vi "RP Read Subset.vi"(6 "Mode":T2=enum."Digitizer", 8 "Error In":errorcluster, 9 "Parameters":T1={"Ranges"=[20.0, 20.0], "Output frequency 1"=50000.0, "Output frequency 2"=50000.0, "Trigger offset"=-100000, "Post-trigger samples"=11534336, "Desimation rate"=125} {"Post-trigger samples" format="0x%x (%d)"; "Trigger offset" format="0x%x (%d)"; "Output frequency 2" format="%#_6p"; "Output frequency 1" format="%#_6p"}, 11 "connection ID":refnum<k5>) -> (0 "Error Out":errorcluster, 1 "Record start pos":u32=1, 2 "Data stream":string, 3 "connection ID out":refnum<k5>)   [LabVIEW 2015]
uses:
  Mode.ctl
  Red Pitaya Parameters.ctl
  RP Command.ctl
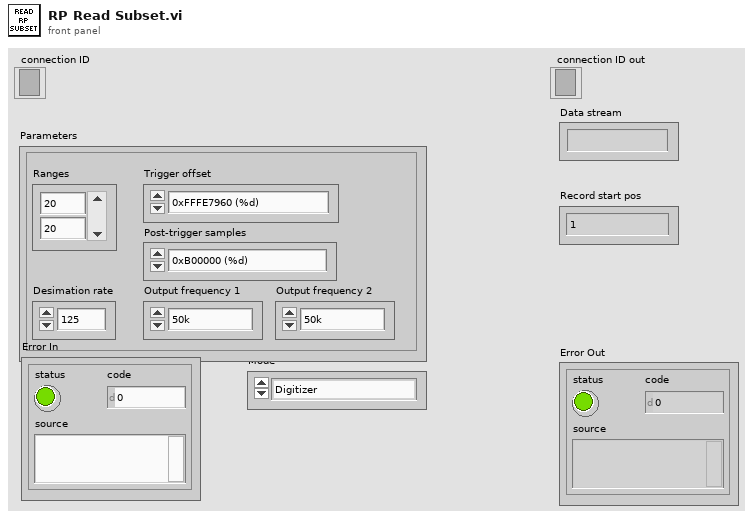
[diagram p1: front panel]
types:
  T1 = typedef "Red Pitaya Parameters.ctl" = cluster{"Ranges":dbl[], "Output frequency 1":dbl, "Output frequency 2":dbl, "Trigger offset":i32, "Post-trigger samples":u64, "Desimation rate":u64}
  T2 = typedef "Mode.ctl" = enum16{"Filter", "Lockin test", "Snapshot test", "Digitizer"}
  T3 = typedef "RP Command.ctl" = enum16{"Set frequency", "Arm and get data", "Stop server", "Get status", "Get temperature", "Set decimation", "Arm", "Software trigger", "Get whole buffer", "Get chunk", "System call", "Get config", "Set config"}
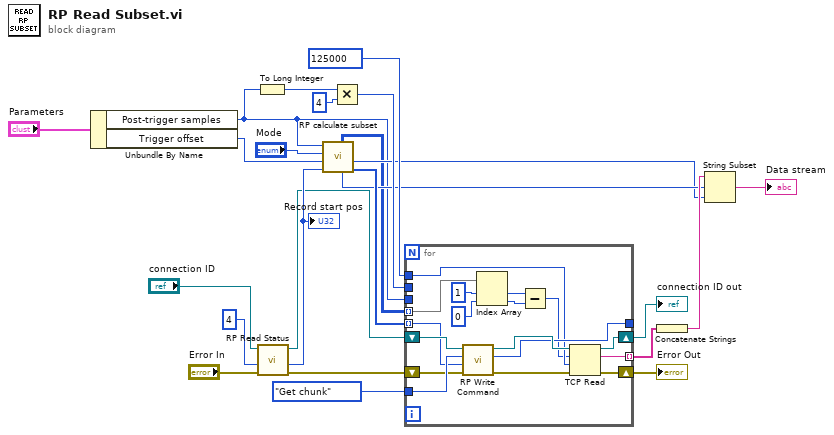
[diagram p0: block diagram]
diagram:
  n1 = Unbundle By Name("Parameters") -> ("Post-trigger samples"=w9:u64, "Trigger offset"=w8:i32)
  n2 = To Long Integer(number=w9) -> (32bit integer=w21:i32)
  n3 = call "RP Read Status.vi"("Error In"="Error In", "Status offset"=u64 4, "connection ID"="connection ID") -> ("Error Out"=w4:errorcluster, "Status response"=w18:u32, "connection ID out"=w17:refnum<k5>)  [unwired: 6 in]
  "Record start pos" <- w18
  n4 = call "RP calculate subset.vi"("Record start position"=w18, "Trigger offset"=w8, "Mode"="Mode", "Post-trigger samples"=w9) -> ("Merged subsets"=w16:u64[], "record length"=w12:i32, "pre-trigger trim"=w13:i32, "Subsets"=w11:i32[][])  [unwired: 2 in, 2 out]
  n5 = Multiply(x=w21, y=4) -> (x*y=w23:i32)
  n6 = for {
    tunnel: w23 -> [_]
    tunnel: RP_Command."Get chunk" ("Command number") -> [w41]
    tunnel: [w38] -> _
    tunnel: 125000 ("timeout ms (25000)") -> [w36]
    tunnel: w9 -> [_]
    shift-right: [w35] -> w2
    shift-left: w4 -> [w34]
    shift-right: [w37] -> w5
    shift-left: w17 -> [w33]
    tunnel: w16 -> [w32] mode=indexing
    tunnel: [w31] -> w15 mode=indexing
    tunnel: w11 -> [w29] mode=indexing
    n7 = call "RP Write Command.vi"("Error In"=w34, "Command payload"=w32, "Command number"=w41, "connection ID"=w33) -> ("Error Out"=w39:errorcluster, "bytes written"=w38:i32, "connection ID out"=w40:refnum<k5>)  [unwired: 5 in]
    n8 = Index Array(array=w29, index #1=1 ("index"), index #2=0 ("index")) -> (element #1=w28:i32, element #2=w27:i32)
    n9 = Subtract(x=w28, y=w27) -> (x-y=w26:i32)
    n10 = TCP Read(connection ID=w40, bytes to read=w26, error in (no error)=w39, 9:w36) -> (connection ID out=w37:refnum<k5>, data out=w31:string, error out=w35:errorcluster)  [unwired: 1 in]
  }
  "connection ID out" <- w5
  "Error Out" <- w2
  n11 = Concatenate Strings(w15) -> (w14:string)
  n12 = String Subset(string=w14, offset (0)=w13, length (rest)=w12) -> (substring=→"Data stream":string)
